vi "WXA100-06MH.vi"() -> ()   [LabVIEW 2016, in "AIRMAR WeatherCaster.lvlib"]
uses:
  AIRMAR WeatherCaster.lvlib
  <vilib>/Utility/miscctls.llb/LVPointTypeDef.ctl
  <vilib>/Plasmionique/MB Master/MB_Master_Serial/MB_Master_Serial.lvclass
  C:/Program Files (x86)/National Instruments/LabVIEW 2016/vi.lib/Plasmionique/MB Master/MB_Master/MB_Master.lvclass
  <vilib>/Instr/_visa.llb/VISA Configure Serial Port (Instr).vi
  <vilib>/Plasmionique/MB Master/MB Master.lvlib
panel:
  in  "风向校准":bool
  out "当前时间":timestamp
  out "通信 2":bool caption="通信"
  in  "校准角度":dbl caption="纠偏角" format="%#.2g"
  in  "电子罗盘配置":T1={"VISA resource name"="", "baud rate (9600)"=9600, "串口打开"=FALSE} {"baud rate (9600)" items=["1200"=1200, "2400"=2400, "4800"=4800, "9600"=9600, "38400"=38400, "115200"=115200]}
  out "电子罗盘角度":T2 scale=0.0..360.0
  out "湿度":dbl format="%#.2g"
  out "data":T3
  out "通信":bool
  in  "串口打开":bool
  in  "baud rate (9600)":u32(ring)=4800 caption="波特率" items=["1200"=1200, "2400"=2400, "4800"=4800, "9600"=9600, "38400"=38400, "115200"=115200]
  in  "VISA resource name":refnum<visa-resource-name> caption="串口"
  out "风向_真角":dbl caption="风向" format="%#.2g"
  out "风速_m/s":dbl caption="风速" format="%#.2g"
  out "气温_摄氏度":dbl caption="气温" format="%#.2g"
  out "气压_bars":dbl caption="气压" format="%#.2g"
  # "%RH"
  # "°"
  # "m/s"
  # "℃"
  # "mbars"
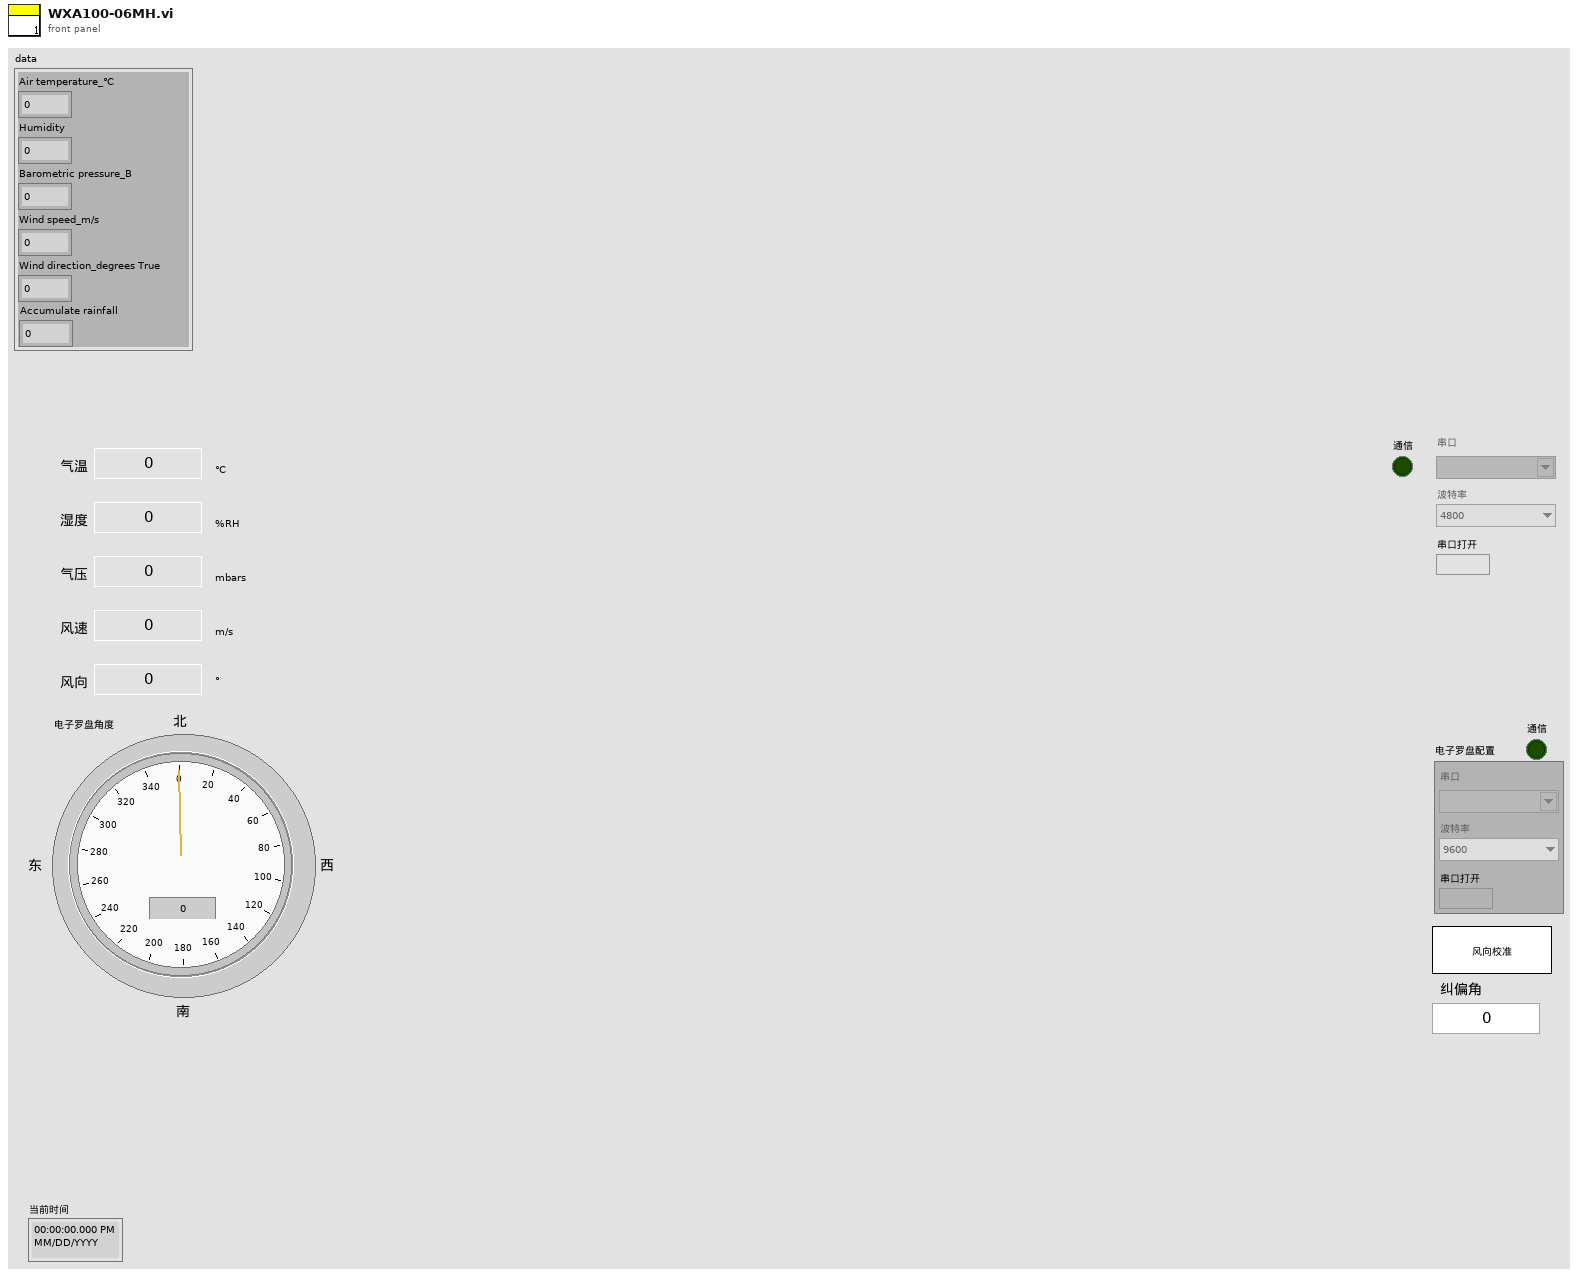
[diagram p1: front panel]
types:
  T1 = cluster{"VISA resource name":refnum<visa-resource-name>, "baud rate (9600)":u32, "串口打开":bool}
  T2 = typedef "电子罗盘.ctl" = dbl
  T3 = cluster{"Air temperature_℃":sgl, "Humidity":sgl, "Barometric pressure_B":sgl, "Wind speed_m/s":sgl, "Wind direction_degrees True":sgl, "Accumulate rainfall":sgl}
  T4 = typedef "LVPointTypeDef.ctl" = cluster{"Horizontal":i16, "Vertical":i16}
  T5 = typedef "LVDateTimeRec.ctl" = cluster{"秒数的小数部分":dbl, "秒":i32, "分":i32, "时":i32, "日":i32, "月":i32, "年":i32, "天数（周）":i32, "天数（年）":i32, "DST":i32}
  T6 = enum8{"Enabled", "Disabled", "Disabled and Grayed Out"}
  T7 = cluster{"baud rate (bps)":u32, "stop bits":u16, "parity":u16, "flow control":u16, "timeout":u32, "retries":i32}
  T8 = cluster{"FLOAT[0]":sgl, "FLOAT[1]":sgl, "FLOAT[2]":sgl, "FLOAT[3]":sgl, "FLOAT[4]":sgl, "FLOAT[5]":sgl}
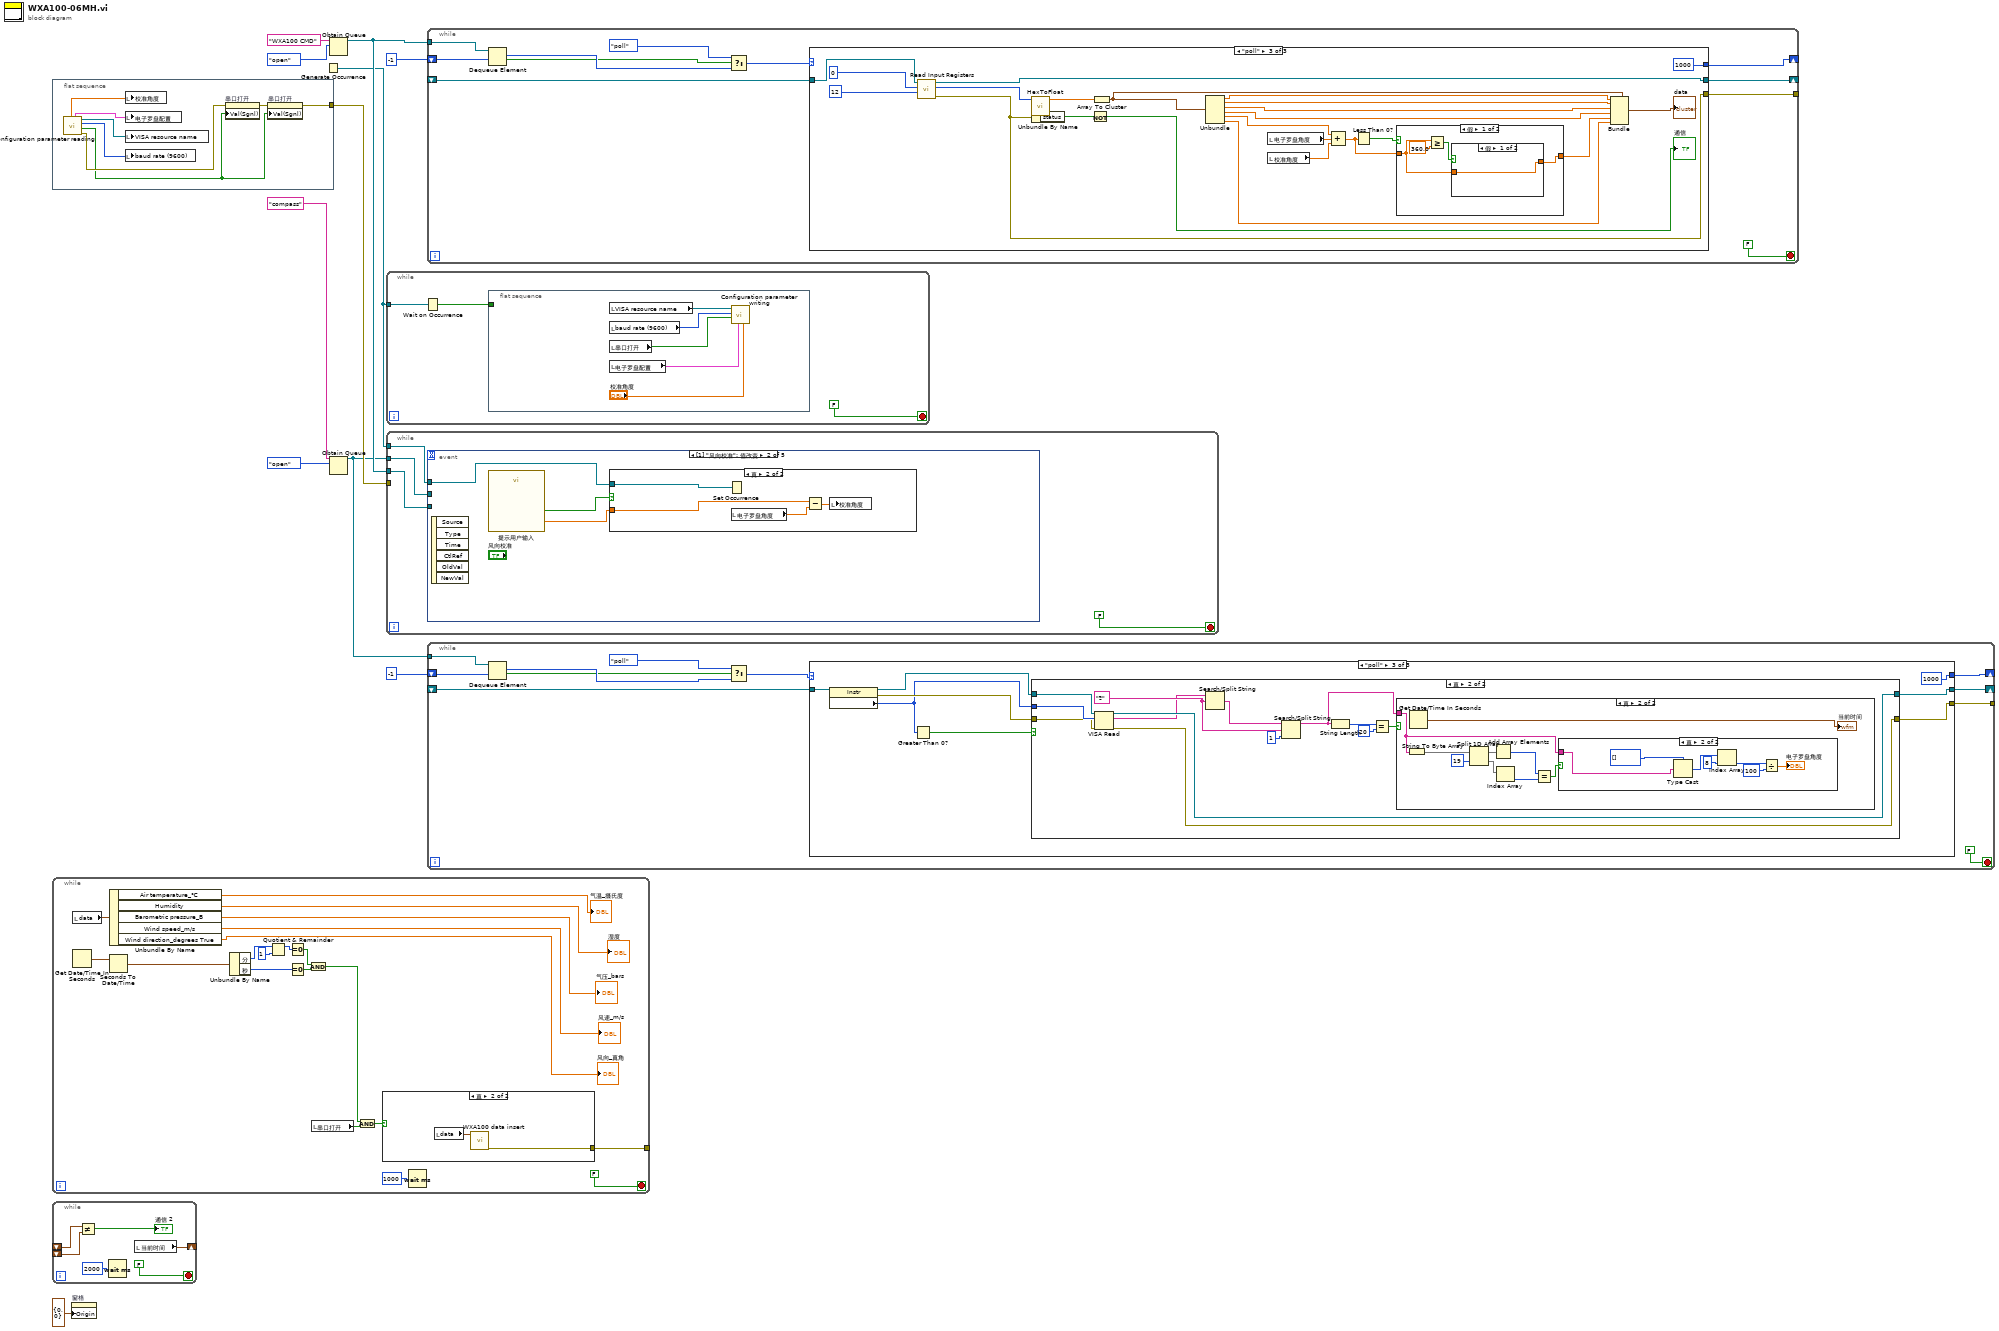
[diagram p0: block diagram]
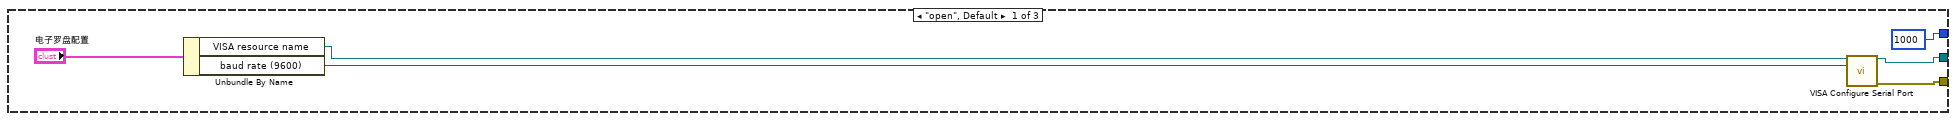
[diagram p2: hidden frame]
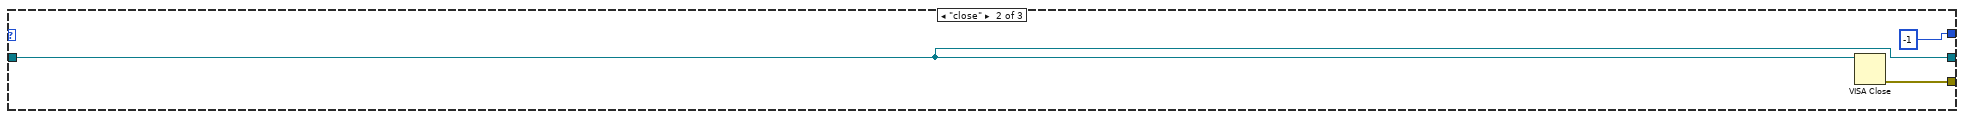
[diagram p3: hidden frame]
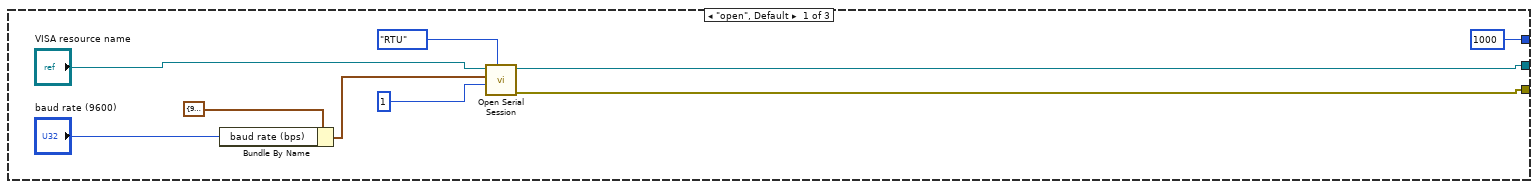
[diagram p8: hidden frame]
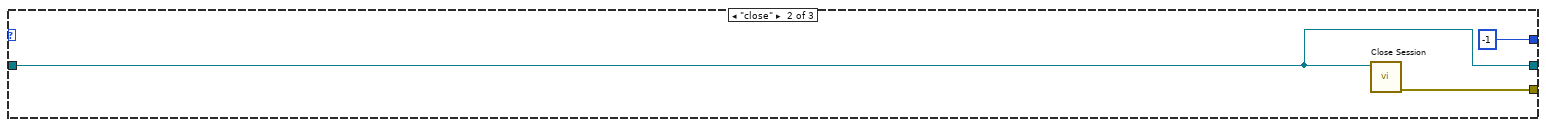
[diagram p9: hidden frame]
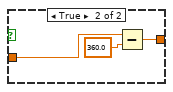
[diagram p10: hidden frame]
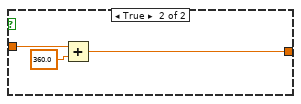
[diagram p11: hidden frame]
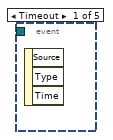
[diagram p12: hidden frame]
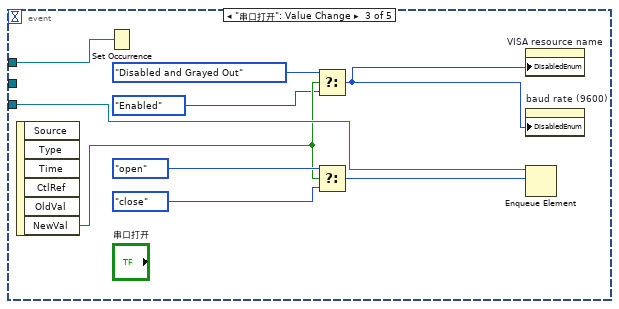
[diagram p14: hidden frame]
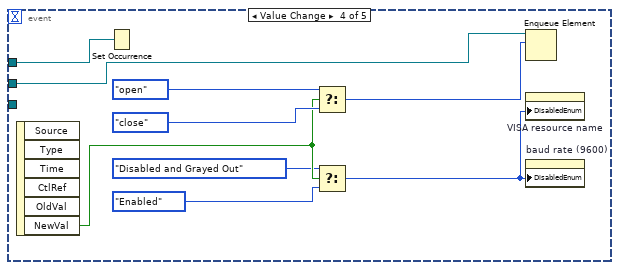
[diagram p15: hidden frame]
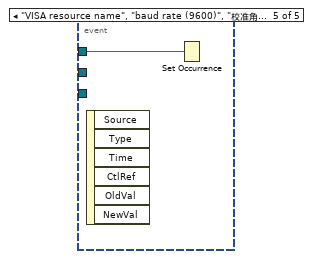
[diagram p16: hidden frame]
diagram:
  n1 = flat-sequence {
    tunnel: [w13] -> w7
    frame #0 {
      n2 = call "Configuration parameter reading.vi"() -> ("error out"=w19:errorcluster, "enable"=w12:bool, "baud rate (9600)"=w17:u32, "VISA resource name"=w18:refnum<visa-resource-name>, "电子罗盘"=w16:T1, "Calibration angle"=w15:sgl)  [unwired: 5 in, 1 out]
      n3 = local write "校准角度"(w15) -> ()
      n4 = local write "电子罗盘配置"(w16) -> ()
      n5 = local write "VISA resource name"(w18) -> ()
      n6 = local write "baud rate (9600)"(w17) -> ()
      n7 = property on="串口打开" class="Bool (严格)"(error in=w19, "Val(Sgnl)"=w12) -> (error out=w14:errorcluster)  [unwired: 1 in, 1 out]
      n8 = property on="串口打开" class="Bool (严格)"(error in=w14, "Val(Sgnl)"=w12) -> (error out=w13:errorcluster)  [unwired: 1 in, 1 out]
    }
  }
  n9 = while {
    tunnel: [w20] -> _
    stop <- FALSE stop-if-true
    n10 = local read "data"() -> (w38:T3)
    n11 = Get Date/Time In Seconds() -> (seconds since 1Jan1904=w29:timestamp)
    n12 = Unbundle By Name(w38) -> ("Air temperature_℃"=→"气温_摄氏度":sgl, "Humidity"=→"湿度":sgl, "Barometric pressure_B"=→"气压_bars":sgl, "Wind speed_m/s"=→"风速_m/s":sgl, "Wind direction_degrees True"=→"风向_真角":sgl)
    n13 = Seconds To Date/Time(time stamp (now)=w29) -> (date time rec=w21:T5)  [unwired: 1 in]
    n14 = Unbundle By Name(w21) -> ("分"=w22:i32, "秒"=w25:i32)
    n15 = Quotient & Remainder(x=w22, y=1) -> (x-y*floor(x/y)=w24:i32)  [unwired: 1 out]
    n16 = Equal To 0?(x=w24) -> (x = 0?=w26:bool)
    n17 = Equal To 0?(x=w25) -> (x = 0?=w27:bool)
    n18 = And(x=w26, y=w27) -> (x .and. y?=w28:bool)
    n19 = local read "串口打开"() -> (w31:bool)
    n20 = And(x=w28, y=w31) -> (x .and. y?=w30:bool)
    n21 = case shown="真" w30 {
      tunnel: [_ w41] -> w20
      frame False {
      }
      frame True {
        n22 = local read "data"() -> (w40:T3)
        n23 = call "WXA100 data insert.vi"("data"=w40) -> ("error out"=w41:errorcluster)  [unwired: 10 in]
      }
    }
    n24 = Wait (ms)(milliseconds to wait=u32 1000 ("等待时间（毫秒）")) -> ()  [unwired: 1 out]
  }
  n25 = while {
    shift-right: [w45] -> _
    shift-left: _ -> [w44]
    shift-left: _ -> [w43]
    stop <- FALSE stop-if-true
    n26 = Not Equal?(x=w44, y=w43) -> (x != y?=→"通信 2":bool)
    n27 = Wait (ms)(milliseconds to wait=u32 2000 ("等待时间（毫秒）")) -> ()  [unwired: 1 out]
    n28 = local read "当前时间"() -> (w45:timestamp)
  }
  n29 = property on="窗格" class="Pane"("Origin"=T4 {"Horizontal"=0, "Vertical"=0} ("原点")) -> ()  [unwired: 2 in, 2 out]
  n30 = Generate Occurrence() -> (w6:refnum<k4>)
  n31 = Obtain Queue(name (unnamed)="WXA100 CMD" ("名称（未命名）"), element data type=enum16{"open", "close", "poll"}."open" ("枚举")) -> (queue out=w9:refnum<queue>)  [unwired: 3 in, 2 out]
  n32 = Obtain Queue(name (unnamed)="compass" ("名称（未命名）"), element data type=enum16{"open", "close", "poll"}."open" ("枚举")) -> (queue out=w1:refnum<queue>)  [unwired: 3 in, 2 out]
  n33 = while {
    tunnel: w6 -> [w50]
    stop <- FALSE stop-if-true
    n34 = Wait on Occurrence(2:w50) -> (0:w49:bool)  [unwired: 2 in]
    n35 = flat-sequence {
      tunnel: w49 -> [_]
      frame #0 {
        n36 = local read "VISA resource name"() -> (w55:refnum<visa-resource-name>)
        n37 = local read "baud rate (9600)"() -> (w54:u32)
        n38 = local read "串口打开"() -> (w53:bool)
        n39 = local read "电子罗盘配置"() -> (w52:T1)
        n40 = call "Configuration parameter writing.vi"("Calibration angle"="校准角度", "电子罗盘"=w52, "enable"=w53, "baud rate (9600)"=w54, "VISA resource name"=w55) -> ()  [unwired: 6 in, 1 out]
      }
    }
  }
  n41 = while {
    tunnel: w9 -> [w58]
    tunnel: w7 -> [_]
    tunnel: w6 -> [w57]
    tunnel: w1 -> [w56]
    stop <- FALSE stop-if-true
    n42 = event shown="[1] \"风向校准\": 值改变" {
      selector: _ -> [_ _ _ _ _]
      dyn-events: _ -> [_ _ _ _ _]
      timeout: _ -> [_ _ _ _ _]
      tunnel: w58 -> [_ _ w72 _ _]
      tunnel: w57 -> [_ w60 w71 w81 w85]
      tunnel: w56 -> [_ _ _ w76 _]
      event Timeout {
        n43 = event-data() -> ()  [unwired: 1 in, 3 out]
      }
      event "风向校准": Value Change {
        n44 = event-data() -> ()  [unwired: 1 in, 6 out]
        n45 = call "提示用户输入"() -> ("角度"=w62:dbl, "确定"=w61:bool)  [unwired: 17 in, 1 out]
        n46 = case shown="真" w61 {
          tunnel: w62 -> [_ w66]
          tunnel: w60 -> [_ w63]
          frame False {
          }
          frame True {
            n47 = Set Occurrence(w63) -> ()
            n48 = local read "电子罗盘角度"() -> (w65:T2)
            n49 = Subtract(x=w66, y=w65) -> (x-y=w64:T2)
            n50 = local write "校准角度"(w64) -> ()
          }
        }
      }
      event "串口打开": Value Change {
        n51 = event-data() -> ("NewVal"=w70:bool)  [unwired: 1 in, 5 out]
        n52 = Set Occurrence(w71) -> ()
        n53 = Select(t=T6."Disabled and Grayed Out" ("禁用"), s=w70, f=T6."Enabled" ("禁用")) -> (s? t:f=w67:T6)
        n54 = Select(t=enum16{"open", "close", "poll"}."open" ("元素"), s=w70, f=enum16{"open", "close", "poll"}."close") -> (s? t:f=w74:enum16{"open", "close", "poll"})
        n55 = property on="VISA resource name" class="VISAName"("DisabledEnum"=w67) -> ()  [unwired: 2 in, 2 out]
        n56 = property on="baud rate (9600)" class="Ring (严格)"("DisabledEnum"=w67) -> ()  [unwired: 2 in, 2 out]
        n57 = Enqueue Element(queue=w72, element=w74) -> ()  [unwired: 2 in, 3 out]
      }
      event "电子罗盘配置.串口打开": Value Change {
        n58 = event-data() -> ("NewVal"=w80:bool)  [unwired: 1 in, 5 out]
        n59 = Set Occurrence(w81) -> ()
        n60 = Select(t=enum16{"open", "close", "poll"}."open" ("元素"), s=w80, f=enum16{"open", "close", "poll"}."close") -> (s? t:f=w83:enum16{"open", "close", "poll"})
        n61 = Select(t=T6."Disabled and Grayed Out" ("禁用"), s=w80, f=T6."Enabled" ("禁用")) -> (s? t:f=w77:T6)
        n62 = Enqueue Element(queue=w76, element=w83) -> ()  [unwired: 2 in, 3 out]
        n63 = property on="VISA resource name" class="VISAName"("DisabledEnum"=w77) -> ()  [unwired: 2 in, 2 out]
        n64 = property on="baud rate (9600)" class="Ring (严格)"("DisabledEnum"=w77) -> ()  [unwired: 2 in, 2 out]
      }
      event "VISA resource name", "baud rate (9600)", "电子罗盘配置.VISA resource name", "电子罗盘配置.baud rate (9600)", "校准角度": Value Change {
        n65 = event-data() -> ()  [unwired: 1 in, 6 out]
        n66 = Set Occurrence(w85) -> ()
      }
    }
  }
  n67 = while {
    tunnel: w9 -> [w96]
    shift-right: [w86] -> _
    shift-left: -1 ("超时毫秒(-1)") -> [w95]
    shift-right: [w90] -> _
    shift-left: _ -> [w88]
    tunnel: [w89] -> _
    stop <- FALSE stop-if-true
    n68 = Dequeue Element(queue=w96, timeout in ms (-1)=w95) -> (element=w93:enum16{"open", "close", "poll"}, timed out?=w92:bool)  [unwired: 1 in, 2 out]
    n69 = Select(t=enum16{"open", "close", "poll"}."poll" ("枚举"), s=w92, f=w93) -> (s? t:f=w91:enum16{"open", "close", "poll"})
    n70 = case shown="\"poll\"" w91 {
      tunnel: [w99 w107 w127] -> w90
      tunnel: [w98 w108 w126] -> w89
      tunnel: w88 -> [_ w107 w131]
      tunnel: [1000 ("超时毫秒(-1)") -1 ("超时毫秒(-1)") 1000 ("超时毫秒(-1)")] -> w86
      frame "open", Default {
        n71 = Bundle By Name(cluster=T7 {"baud rate (bps)"=9600, "stop bits"=10, "parity"=0, "flow control"=0, "timeout"=1000, "retries"=1} ("Serial Config"), "baud rate (bps)"="baud rate (9600)") -> (w101:T7)
        n72 = call <vilib>:"Open Serial Session.vi"("Mode (RTU)"=enum16{"RTU", "ASCII"}."RTU", "Slave ID"=u8 1, "Serial Config"=w101, "VISA Resource"="VISA resource name") -> ("Error out"=w98:errorcluster, "MB_Serial session"=w99:refnum<class "MB_Master_Serial.lvclass">)  [unwired: 6 in]
      }
      frame "close" {
        n73 = call-dynamic "Close Session.vi"("MB_Serial session"=w107) -> ("error out"=w108:errorcluster)  [unwired: 10 in]
      }
      frame "poll" {
        n74 = call <vilib>:"Read Input Registers.vi"("quantity"=u16 12, "starting address"=u16 0, "MB session in"=w131) -> ("error out"=w126:errorcluster, "Registers"=w128:u16[], "MB session out"=w127:refnum<class "MB_Master_Serial.lvclass">)  [unwired: 6 in]
        n75 = call "HexToFloat.vi"("数组"=w128) -> ("FLOAT"=w123:sgl[])  [unwired: 10 in]
        n76 = Unbundle By Name(w126) -> ("status"=w125:bool)
        n77 = Not(x=w125) -> (.not. x?=→"通信":bool)
        n78 = Array To Cluster(array=w123) -> (cluster=w121:T8)
        n79 = Unbundle(w121) -> ("FLOAT[0]"=w119:sgl, "FLOAT[1]"=w118:sgl, "FLOAT[2]"=w117:sgl, "FLOAT[3]"=w116:sgl, "FLOAT[4]"=w114:sgl, "FLOAT[5]"=w115:sgl)
        n80 = local read "电子罗盘角度"() -> (w110:T2)
        n81 = local read "校准角度"() -> (w109:dbl)
        n82 = Compound Arithmetic op=ADD(w114, w110, w109) -> (w113:T2)
        n83 = Less Than 0?(x=w113) -> (x < 0?=w112:bool)
        n84 = case shown="假" w112 {
          tunnel: w113 -> [w133 w142]
          tunnel: [w132 w140] -> w111
          frame False {
            n85 = Greater Or Equal?(x=w133, y=T2 360.0) -> (x >= y?=w134:bool)
            n86 = case shown="假" w134 {
              tunnel: w133 -> [w136 w139]
              tunnel: [w136 w137] -> w132
              frame False {
              }
              frame True {
                n87 = Subtract(x=w139, y=T2 360.0) -> (x-y=w137:T2)
              }
            }
          }
          frame True {
            n88 = Add(x=w142, y=360.0) -> (x+y=w140:T2)
          }
        }
        n89 = Bundle(cluster=w121, "FLOAT[0]"=w119, "FLOAT[1]"=w118, "FLOAT[2]"=w117, "FLOAT[3]"=w116, "FLOAT[4]"=w111, "FLOAT[5]"=w115) -> (→"data":T8)
      }
    }
  }
  n90 = while {
    tunnel: w1 -> [w153]
    shift-right: [w145] -> _
    shift-left: -1 ("超时毫秒(-1)") -> [w152]
    tunnel: [w147] -> _
    shift-right: [w144] -> _
    shift-left: _ -> [w143]
    stop <- FALSE stop-if-true
    n91 = Dequeue Element(queue=w153, timeout in ms (-1)=w152) -> (element=w150:enum16{"open", "close", "poll"}, timed out?=w149:bool)  [unwired: 1 in, 2 out]
    n92 = Select(t=enum16{"open", "close", "poll"}."poll" ("枚举"), s=w149, f=w150) -> (s? t:f=w148:enum16{"open", "close", "poll"})
    n93 = case shown="\"poll\"" w148 {
      tunnel: [w154 w161 w164] -> w147
      tunnel: [1000 ("超时毫秒(-1)") -1 ("超时毫秒(-1)") 1000 ("超时毫秒(-1)")] -> w145
      tunnel: [w155 w160 w163] -> w144
      tunnel: w143 -> [_ w160 w168]
      frame "open", Default {
        n94 = Unbundle By Name("电子罗盘配置") -> ("VISA resource name"=w157:refnum<visa-resource-name>, "baud rate (9600)"=w156:u32)
        n95 = call-poly "VISA Configure Serial Port"("VISA resource name"=w157, "baud rate (9600)"=w156) -> ("VISA resource name out"=w155:refnum<visa-resource-name>, "error out"=w154:errorcluster)  [unwired: 12 in]
      }
      frame "close" {
        n96 = VISA Close(VISA resource name=w160) -> (error out=w161:errorcluster)  [unwired: 1 in]
      }
      frame "poll" {
        n97 = property class="Instr"(reference=w168) -> (reference out=w167:refnum<visa-resource-name>, error out=w166:errorcluster, "Serial Settings:Number of Bytes at Serial Port"=w165:u32)  [unwired: 1 in]
        n98 = Greater Than 0?(x=w165) -> (x > 0?=w169:bool)
        n99 = case shown="真" w169 {
          tunnel: w167 -> [w172 w185]
          tunnel: [w172 w184] -> w163
          tunnel: [w171 w183] -> w164
          tunnel: w166 -> [w171 w181]
          tunnel: w165 -> [_ w182]
          frame False {
          }
          frame True {
            w179 = "ª" ("正则表达式")
            n100 = VISA Read(VISA resource name=w185, byte count=w182, error in (no error)=w181) -> (VISA resource name out=w184:refnum<visa-resource-name>, read buffer=w173:string, error out=w183:errorcluster)  [unwired: 1 out]
            n101 = Search/Split String(string=w173, search string/char (-)=w179) -> (match + rest of string=w180:string)  [unwired: 1 in, 2 out]
            n102 = Search/Split String(string=w180, search string/char (-)=w179, offset (0)=1 ("偏移量(0)")) -> (substring before match=w174:string)  [unwired: 2 out]
            n103 = String Length(string=w174) -> (length=w178:i32)
            n104 = Equal?(x=w178, y=20) -> (x = y?=w175:bool)
            n105 = case shown="真" w175 {
              tunnel: w174 -> [_ w194]
              frame False {
              }
              frame True {
                n106 = String To Byte Array(string=w194) -> (unsigned byte array=w193:u8[])
                n107 = Get Date/Time In Seconds() -> (seconds since 1Jan1904=→"当前时间":timestamp)
                n108 = Split 1D Array(array=w193, index=19 ("索引")) -> (first subarray=w191:u8[], second subarray=w190:u8[])
                n109 = Add Array Elements(numeric array=w191) -> (sum=w188:u8)
                n110 = Index Array(array=w190) -> (element=w189:u8)  [unwired: 1 in]
                n111 = Equal?(x=w188, y=w189) -> (x = y?=w187:bool)
                n112 = case shown="真" w187 {
                  tunnel: w194 -> [_ w196]
                  frame False {
                  }
                  frame True {
                    n113 = Type Cast(type=u16[] [], x=w196) -> (*(type *) &x=w199:u16[])
                    n114 = Index Array(array=w199, index=8 ("索引")) -> (element=w198:u16)
                    n115 = Divide(x=w198, y=u16 100) -> (x/y=→"电子罗盘角度":dbl)
                  }
                }
              }
            }
          }
        }
      }
    }
  }
